vi "Flatten.vi"(8 "error in (no error)":errorcluster, 11 "Scanner in":refnum<class "Scanner.lvclass">) -> (0 "error out":errorcluster, 3 "Scanner out":refnum<class "Scanner.lvclass">)   [LabVIEW 2015, in "Scanner.lvclass"]
uses:
  Scanner.lvclass
  Scanner.lvclass/Scanner.ctl
  Global/File Locations.vi
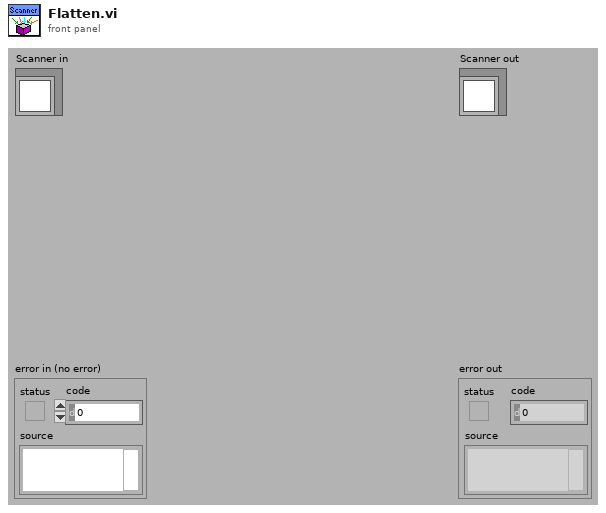
[diagram p1: front panel]
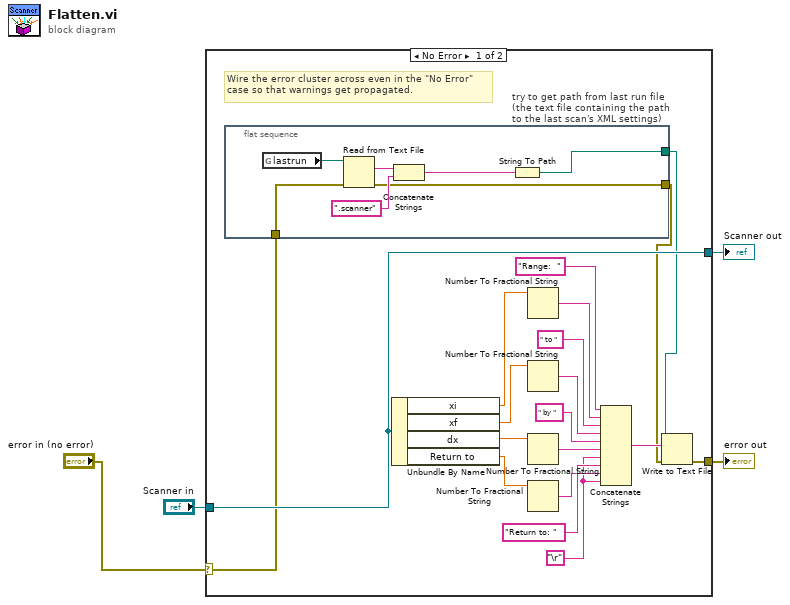
[diagram p0: block diagram]
diagram:
  n1 = case shown="No Error" "error in (no error)" {
    selector: "error in (no error)" -> [w7 w31]
    tunnel: [w22 w31] -> w4
    tunnel: [w23 w32] -> w2
    tunnel: "Scanner in" -> [w23 w32]
    frame No Error {
      w8 = "\r"
      # "Wire the error cluster across even in the \"No Error\"\ncase so that warnings get propagated."
      n2 = flat-sequence "try to get path from last run file\n(the text file containing the path\nto the last scan's XML settings)" {
        tunnel: [w24] -> w6
        tunnel: [w26] -> w5
        tunnel: w7 -> [w25]
        frame #0 {
          n3 = global read "File Locations.vi" "lastrun"() -> (w30:path)
          n4 = Read from Text File(file (use dialog)=w30, error in=w25) -> (text=w29:string, error out=w24:errorcluster)  [unwired: 4 out]
          n5 = Concatenate Strings(w29, ".scanner") -> (w27:string)
          n6 = String To Path(string=w27) -> (path=w26:path)
        }
      }
      n7 = Unbundle By Name(w23) -> ("xi"=w19:dbl, "xf"=w16:dbl, "dx"=w11:dbl, "Return to"=w10:dbl)
      n8 = Number To Fractional String(number=w19) -> (F-format string=w18:string)  [unwired: 3 in]
      n9 = Number To Fractional String(number=w16) -> (F-format string=w15:string)  [unwired: 3 in]
      n10 = Number To Fractional String(number=w11) -> (F-format string=w13:string)  [unwired: 3 in]
      n11 = Number To Fractional String(number=w10) -> (F-format string=w9:string)  [unwired: 3 in]
      n12 = Concatenate Strings("Range:  ", w18, " to ", w15, " by ", w13, w8, "Return to: ", w9, w8) -> (w21:string)
      n13 = Write to Text File(file (use dialog)=w5, text=w21, error in=w6) -> (error out=w22:errorcluster)  [unwired: 1 in, 2 out]
    }
    frame Error {
    }
  }
  "error out" <- w4
  "Scanner out" <- w2
